vi "Stop Core.vi"(10 "final error code":i32, 11 "Sequencer in":refnum<class "Sequencer.lvclass">) -> (3 "Sequencer out":refnum<class "Sequencer.lvclass">)   [LabVIEW 2020, in "Sequencer.lvlib" / "Sequencer.lvclass"]
doc: "(<B>Filename</B>: Actor Framework.lvlib:Actor.lvclass:Stop Core.vi)\n\nDefines what the actor does before it stops. Use the <B>final error code</B> input to determine whether the actor shut down in response to an error.\n\nThis implementation closes the Core Enqueue Lock semaphore."
uses:
  Sequencer.lvclass
  Sequencer.lvclass/Sequencer.ctl
  PPL/HDH.Actor Framework.Core.Actor.lvlibp/1abvi3w/vi.lib/ActorFramework/Actor/Actor.lvclass
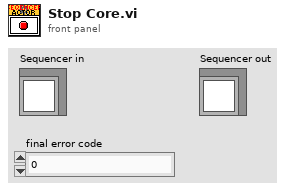
[diagram p1: front panel]
types:
  T1 = typedef "Semaphore RefNum" = refnum<k1>
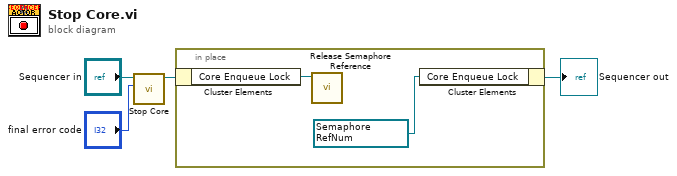
[diagram p0: block diagram]
diagram:
  n1 = call-parent "Stop Core.vi"("final error code"="final error code", "Actor in"="Sequencer in") -> ("Actor out"=w2:refnum<class "Sequencer.lvclass">)  [unwired: 9 in]
  n2 = in-place {
    w5 = T1 refnum items=["semaphore"] ("Core Enqueue Lock")
    n3 = in-place-cluster #1(w2) -> ("Core Enqueue Lock"=w6:T1)
    n4 = call <vilib>:"Release Semaphore Reference.vi"("semaphore"=w6) -> ()  [unwired: 9 in, 2 out]
    n5 = in-place-cluster #1("Core Enqueue Lock"=w5) -> (→"Sequencer out":refnum<class "Sequencer.lvclass">)
  }
